vi "search_relative_path.vi"(8 "error in (no error)":errorcluster, 10 "calling_path":path, 11 "path_relative":path) -> (0 "error out":errorcluster, 2 "file or folder exists?":bool, 3 "path_absolute":path)   [LabVIEW 2015, in "lv-bin.lvlib" / "v1.lvlib"]
uses:
  v1.lvlib
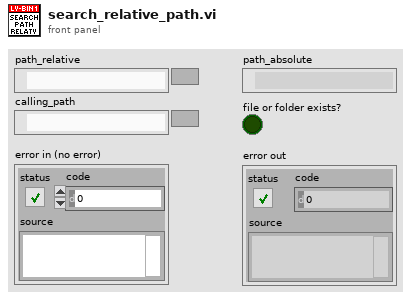
[diagram p1: front panel]
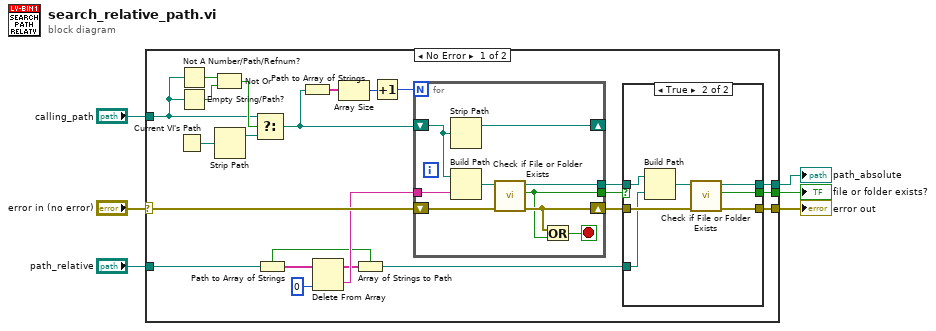
[diagram p0: block diagram]
diagram:
  n1 = case shown="No Error" "error in (no error)" {
    selector: "error in (no error)" -> [w14 w48]
    tunnel: "path_relative" -> [w7 _]
    tunnel: [w28 w48] -> w3
    tunnel: "calling_path" -> [w24 _]
    tunnel: [w21 _] -> w2
    tunnel: [w20 _] -> w1
    frame No Error {
      n2 = Current VI's Path() -> (path=w17:path)
      n3 = Not A Number/Path/Refnum?(number/path/refnum=w24) -> (NaN/Path/Refnum?=w26:bool)
      n4 = Empty String/Path?(string/path=w24) -> (empty?=w27:bool)
      n5 = Not Or(1:w27, 2:w26) -> (0:w25:bool)
      n6 = Strip Path(path=w17) -> (stripped path=w16:path)  [unwired: 1 out]
      n7 = Select(t=w24, s=w25, f=w16) -> (s? t:f=w18:path)
      n8 = Path to Array of Strings(0:w7) -> (1:w8:bool, 2:w13:string[])
      n9 = Path to Array of Strings(0:w18) -> (2:w30:string[])  [unwired: 1 out]
      n10 = Delete From Array(array=w13, index=0) -> (deleted portion=w11:string, array with subset deleted=w10:string[])  [unwired: 1 in]
      n11 = Array Size(array=w30) -> (size(s)=w29:i32)
      n12 = Array of Strings to Path(0:w10, 1:w8) -> (2:w9:path)
      n13 = Increment(x=w29) -> (x+1=w19:i32)
      n14 = for {
        N: w19 -> [_]
        shift-right: [w44] -> _
        shift-left: w18 -> [w41]
        tunnel: [w45] -> w23
        shift-right: [w47] -> w22
        shift-left: w14 -> [w43]
        tunnel: [w40] -> w15
        tunnel: w11 -> [w39]
        stop <- w42 stop-if-true
        n15 = Strip Path(path=w41) -> (stripped path=w44:path)  [unwired: 1 out]
        n16 = Build Path(base path=w41, name or relative path=w39) -> (appended path=w46:path)
        n17 = call <vilib>:"Check if File or Folder Exists.vi"("error in (no error)"=w43, "path"=w46) -> ("error out"=w47:errorcluster, "file or folder exists?"=w45:bool, "dup path"=w40:path)  [unwired: 7 in]
        n18 = Or(x=w47, y=w45) -> (x .or. y?=w42:bool)
      }
      n19 = case shown="True" w23 {
        tunnel: w22 -> [w31 w38]
        tunnel: [w31 w34] -> w28
        tunnel: [_ w36] -> w21
        tunnel: [_ w35] -> w20
        tunnel: w15 -> [_ w33]
        tunnel: w9 -> [_ w32]
        frame False {
        }
        frame True {
          n20 = Build Path(base path=w33, name or relative path=w32) -> (appended path=w37:path)
          n21 = call <vilib>:"Check if File or Folder Exists.vi"("error in (no error)"=w38, "path"=w37) -> ("error out"=w34:errorcluster, "file or folder exists?"=w36:bool, "dup path"=w35:path)  [unwired: 7 in]
        }
      }
    }
    frame Error {
    }
  }
  "path_absolute" <- w1
  "error out" <- w3
  "file or folder exists?" <- w2
